vi "Get VIs.vi"(8 "error in (no error)":errorcluster) -> (0 "error out":errorcluster, 3 "VIs":refnum<vi>[](array[refnum]))   [LabVIEW 2025, in "Tools.lvlib"]
uses:
  Tools.lvlib
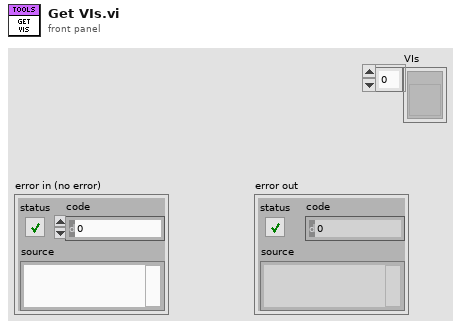
[diagram p1: front panel]
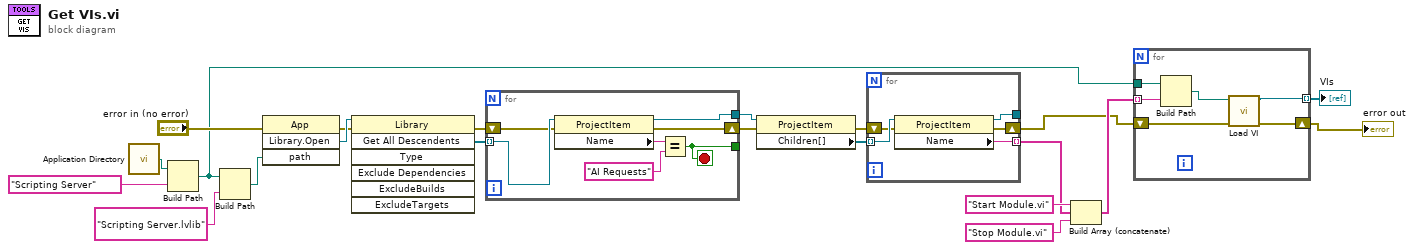
[diagram p0: block diagram]
diagram:
  n1 = call <vilib>:"Application Directory.vi"() -> ("Application Directory"=w15:path)
  n2 = Build Path(base path=w15, name or relative path="Scripting Server" ("format string")) -> (appended path=w1:path)
  n3 = Build Path(base path=w1, name or relative path="Scripting Server.lvlib" ("format string")) -> (appended path=w18:path)
  n4 = invoke class="App" method="Library.Open"(error in="error in (no error)", "path"=w18) -> (error out=w19:errorcluster, "Open Library"=w20:refnum<vi>)  [unwired: 2 in, 2 out]
  n5 = invoke class="Library" method="Get All Descendents"(reference=w20, error in=w19) -> (error out=w12:errorcluster, "All Descendents"=w11:refnum<vi>[])  [unwired: 5 in, 5 out]
  n6 = for {
    tunnel: w11 -> [w28] mode=indexing
    tunnel: [w27] -> w13
    shift-right: [w23] -> w14
    shift-left: w12 -> [w24]
    tunnel: [w22] -> _
    stop <- w22 stop-if-true
    n7 = property class="ProjectItem"(reference=w28, error in=w24) -> (reference out=w27:refnum<vi>, error out=w23:errorcluster, "Name"=w26:string)
    n8 = Equal?(x=w26, y="AI Requests") -> (x = y?=w22:bool)
  }
  n9 = property class="ProjectItem"(reference=w13, error in=w14) -> (error out=w7:errorcluster, "Children[]"=w6:refnum<vi>[])  [unwired: 1 out]
  n10 = for {
    tunnel: w6 -> [w33] mode=indexing
    tunnel: [w32] -> _
    tunnel: [w31] -> w8 mode=indexing
    shift-right: [w29] -> w4
    shift-left: w7 -> [w30]
    n11 = property class="ProjectItem"(reference=w33, error in=w30) -> (reference out=w32:refnum<vi>, error out=w29:errorcluster, "Name"=w31:string)
  }
  n12 = Build Array (concatenate)("Start Module.vi" ("y"), w8, "Stop Module.vi" ("y")) -> (w5:string[])
  n13 = for {
    tunnel: w5 -> [w39] mode=indexing
    shift-right: [w38] -> w3
    shift-left: w4 -> [w37]
    tunnel: [w36] -> w2 mode=indexing
    tunnel: w1 -> [w35]
    n14 = Build Path(base path=w35, name or relative path=w39) -> (appended path=w34:path)
    n15 = call "Load VI.vi"("error in (no error)"=w37, "vi path"=w34) -> ("error out"=w38:errorcluster, "VI out"=w36:refnum<vi>)  [unwired: 8 in]
  }
  "error out" <- w3
  "VIs" <- w2
